vi "SendStatistics.vi"(8 "error in (no error)":errorcluster, 11 "TopLevel in":refnum<class "TopLevel.lvclass">) -> (0 "error out":errorcluster, 3 "TopLevel out":refnum<class "TopLevel.lvclass">)   [LabVIEW 2019, in "TopLevel.lvlib" / "TopLevel.lvclass"]
uses:
  TopLevel.lvclass
  TopLevel.lvclass/TopLevel.ctl
  WebSocket/WebSocket Messages/UpdateStatistics Msg/UpdateStatistics Msg.lvclass/UpdateStatistics Msg.ctl
  <vilib>/ActorFramework/Message Enqueuer/Message Enqueuer.lvclass/Message Enqueuer.ctl
  <vilib>/ActorFramework/Message Enqueuer/Enqueue.vi
  WebSocket/WebSocket Messages/UpdateStatistics Msg/UpdateStatistics Msg.lvclass
  C:/Program Files/National Instruments/LabVIEW 2019/vi.lib/ActorFramework/Message/Message.lvclass
  <vilib>/ActorFramework/Message Priority Queue/Priority Enqueue.vi
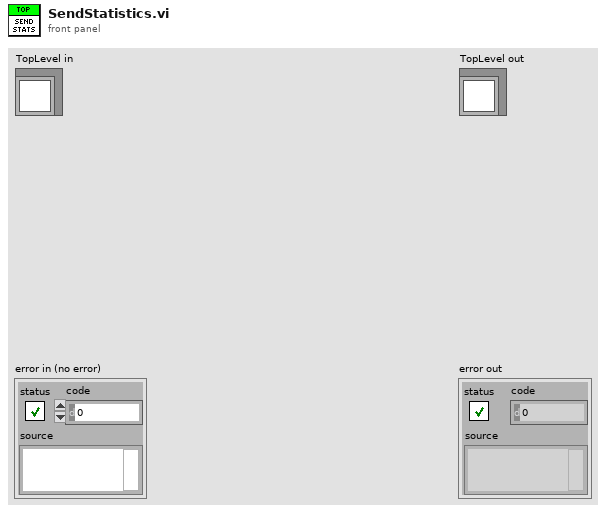
[diagram p1: front panel]
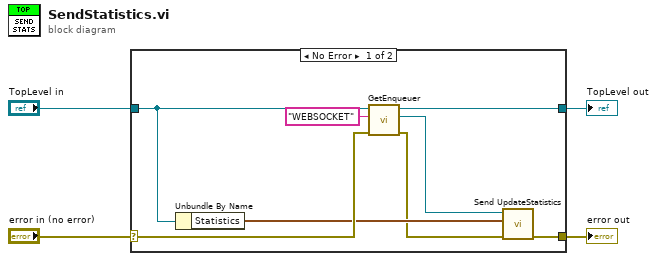
[diagram p0: block diagram]
diagram:
  n1 = case shown="No Error" "error in (no error)" {
    selector: "error in (no error)" -> [w9 w14]
    tunnel: [w6 w14] -> w3
    tunnel: [w10 w13] -> w1
    tunnel: "TopLevel in" -> [w11 w13]
    frame No Error {
      n2 = Unbundle By Name(w11) -> ("Statistics"=w7:cluster{"OK":i32, "NG":i32})
      n3 = call "GetEnqueuer.vi"("error in (no error)"=w9, "Actor Name"="WEBSOCKET", "TopLevel in"=w11) -> ("error out"=w5:errorcluster, "Enqueuer"=w8:refnum<class "Message Enqueuer.lvclass">, "TopLevel out"=w10:refnum<class "TopLevel.lvclass">)  [unwired: 6 in]
      n4 = call "Send UpdateStatistics.vi"("error in (no error)"=w5, "Statistics"=w7, "Message Enqueuer"=w8) -> ("error out"=w6:errorcluster)  [unwired: 7 in, 1 out]
    }
    frame Error {
    }
  }
  "error out" <- w3
  "TopLevel out" <- w1
